vi "PianoTest 8 channel.vi"() -> ()   [LabVIEW 2013]
uses:
  <vilib>/rvi/Emulation/niFpgaSctlEmulationGetInTimedLoop.vi
  <vilib>/rvi/Emulation/niFpgaEmulationReportErrorSimple.vi
  <vilib>/rvi/Emulation/niFpgaGetClockAttributes.vi
  <vilib>/rvi/eio/common/nirviEmuTemplateMethod_errors.vi
  <vilib>/rvi/Emulation/niFpgaCriticalErrorInLSC.vi
  <vilib>/eio/EIONode/EIONode.xnode
panel:
  in  "PWM1 Period (us)":fxp<+/-,20,16>=130.0
  in  "PWM1 Duty Cycle %":fxp<+/-,20,16>=100.0
  in  "Play":bool
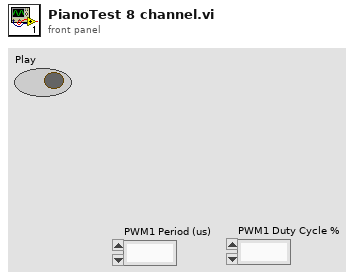
[diagram p1: front panel]
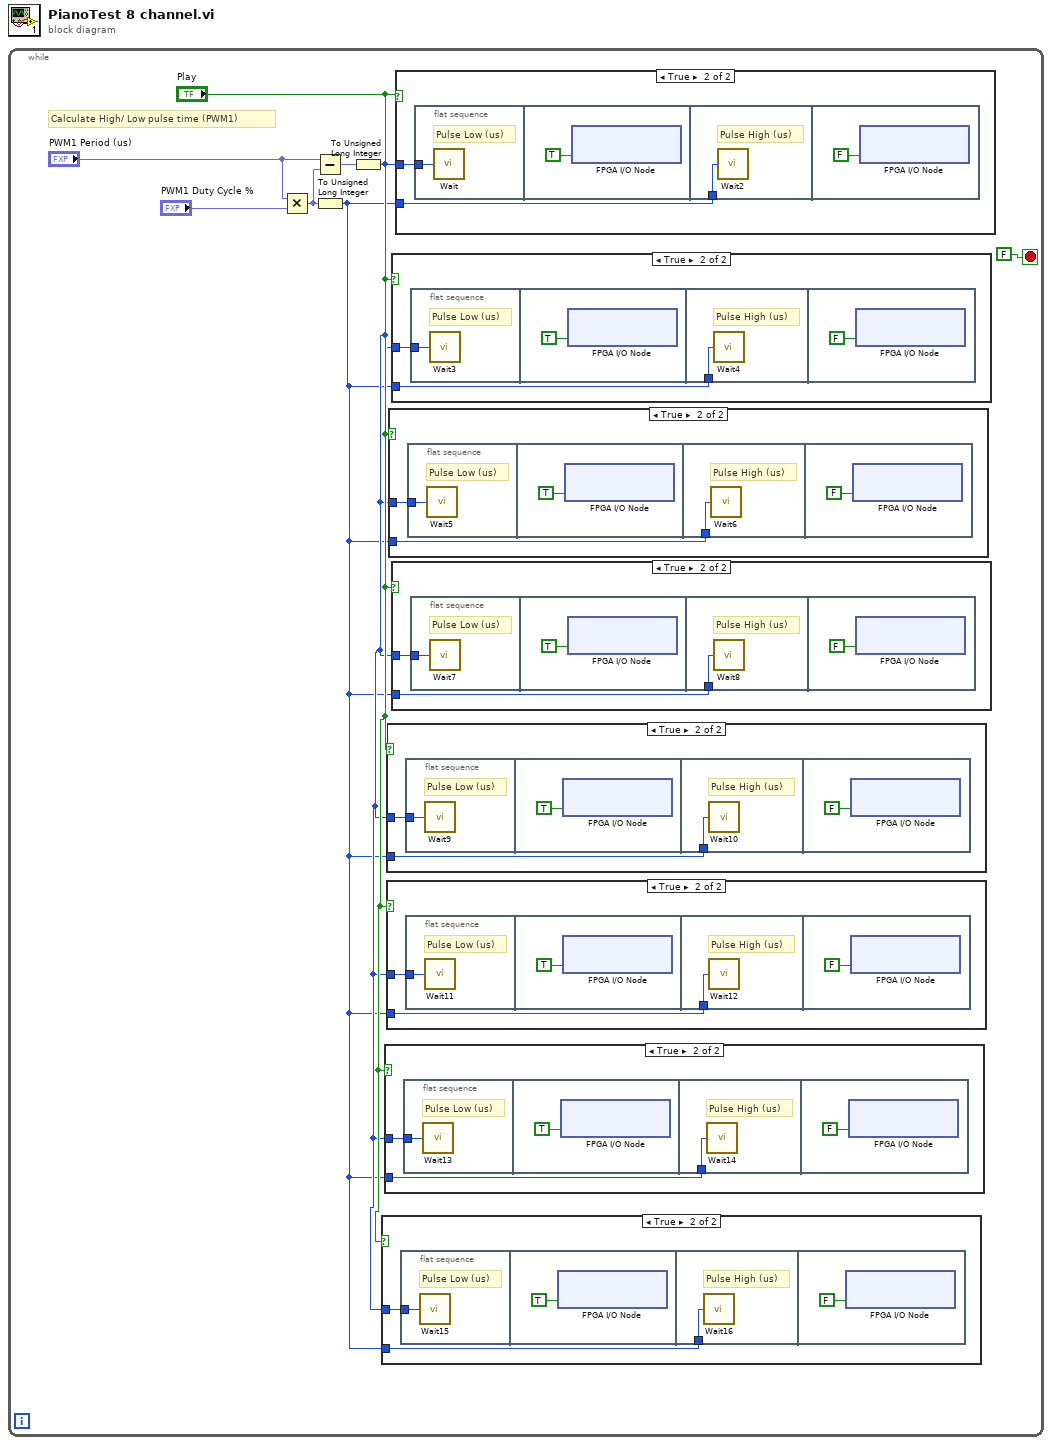
[diagram p0: block diagram]
diagram:
  n1 = while {
    stop <- FALSE stop-if-true
    # "Calculate High/ Low pulse time (PWM1)"
    n2 = Multiply(x="PWM1 Period (us)", y="PWM1 Duty Cycle %") -> (x*y=w7:fxp<+/-,40,32>)
    n3 = Subtract(x="PWM1 Period (us)", y=w7) -> (x-y=w4:fxp<+/-,40,32>)
    n4 = To Unsigned Long Integer(number=w7) -> (unsigned 32bit integer=w1:u32)
    n5 = To Unsigned Long Integer(number=w4) -> (unsigned 32bit integer=w2:u32)
    n6 = case shown="True" "Play" {
      tunnel: w1 -> [_ w10]
      tunnel: w2 -> [_ w9]
      frame False {
      }
      frame True {
        n7 = flat-sequence {
          tunnel: w9 -> [w11]
          tunnel: w10 -> [w13]
          frame #0 {
            # "Pulse Low (us)"
            n8 = call "Wait15"("Count(uSec)"=w11) -> ()  [unwired: 1 out]
          }
          frame #1 {
            n9 = xnode "FPGA I/O Node"("Mod1/DO7"=TRUE ("PWM 1T")) -> ()  [unwired: 1 in, 1 out]
          }
          frame #2 {
            # "Pulse High (us)"
            n10 = call "Wait16"("Count(uSec)"=w13) -> ()  [unwired: 1 out]
          }
          frame #3 {
            n11 = xnode "FPGA I/O Node"("Mod1/DO7"=FALSE ("PWM 1T")) -> ()  [unwired: 1 in, 1 out]
          }
        }
      }
    }
    n12 = case shown="True" "Play" {
      tunnel: w1 -> [_ w16]
      tunnel: w2 -> [_ w15]
      frame False {
      }
      frame True {
        n13 = flat-sequence {
          tunnel: w15 -> [w17]
          tunnel: w16 -> [w19]
          frame #0 {
            # "Pulse Low (us)"
            n14 = call "Wait13"("Count(uSec)"=w17) -> ()  [unwired: 1 out]
          }
          frame #1 {
            n15 = xnode "FPGA I/O Node"("Mod1/DO6"=TRUE ("PWM 1T")) -> ()  [unwired: 1 in, 1 out]
          }
          frame #2 {
            # "Pulse High (us)"
            n16 = call "Wait14"("Count(uSec)"=w19) -> ()  [unwired: 1 out]
          }
          frame #3 {
            n17 = xnode "FPGA I/O Node"("Mod1/DO6"=FALSE ("PWM 1T")) -> ()  [unwired: 1 in, 1 out]
          }
        }
      }
    }
    n18 = case shown="True" "Play" {
      tunnel: w1 -> [_ w28]
      tunnel: w2 -> [_ w27]
      frame False {
      }
      frame True {
        n19 = flat-sequence {
          tunnel: w27 -> [w29]
          tunnel: w28 -> [w31]
          frame #0 {
            # "Pulse Low (us)"
            n20 = call "Wait9"("Count(uSec)"=w29) -> ()  [unwired: 1 out]
          }
          frame #1 {
            n21 = xnode "FPGA I/O Node"("Mod1/DO4"=TRUE ("PWM 1T")) -> ()  [unwired: 1 in, 1 out]
          }
          frame #2 {
            # "Pulse High (us)"
            n22 = call "Wait10"("Count(uSec)"=w31) -> ()  [unwired: 1 out]
          }
          frame #3 {
            n23 = xnode "FPGA I/O Node"("Mod1/DO4"=FALSE ("PWM 1T")) -> ()  [unwired: 1 in, 1 out]
          }
        }
      }
    }
    n24 = case shown="True" "Play" {
      tunnel: w1 -> [_ w22]
      tunnel: w2 -> [_ w21]
      frame False {
      }
      frame True {
        n25 = flat-sequence {
          tunnel: w21 -> [w23]
          tunnel: w22 -> [w25]
          frame #0 {
            # "Pulse Low (us)"
            n26 = call "Wait11"("Count(uSec)"=w23) -> ()  [unwired: 1 out]
          }
          frame #1 {
            n27 = xnode "FPGA I/O Node"("Mod1/DO5"=TRUE ("PWM 1T")) -> ()  [unwired: 1 in, 1 out]
          }
          frame #2 {
            # "Pulse High (us)"
            n28 = call "Wait12"("Count(uSec)"=w25) -> ()  [unwired: 1 out]
          }
          frame #3 {
            n29 = xnode "FPGA I/O Node"("Mod1/DO5"=FALSE ("PWM 1T")) -> ()  [unwired: 1 in, 1 out]
          }
        }
      }
    }
    n30 = case shown="True" "Play" {
      tunnel: w1 -> [_ w40]
      tunnel: w2 -> [_ w39]
      frame False {
      }
      frame True {
        n31 = flat-sequence {
          tunnel: w39 -> [w41]
          tunnel: w40 -> [w43]
          frame #0 {
            # "Pulse Low (us)"
            n32 = call "Wait5"("Count(uSec)"=w41) -> ()  [unwired: 1 out]
          }
          frame #1 {
            n33 = xnode "FPGA I/O Node"("Mod1/DO2"=TRUE ("PWM 1T")) -> ()  [unwired: 1 in, 1 out]
          }
          frame #2 {
            # "Pulse High (us)"
            n34 = call "Wait6"("Count(uSec)"=w43) -> ()  [unwired: 1 out]
          }
          frame #3 {
            n35 = xnode "FPGA I/O Node"("Mod1/DO2"=FALSE ("PWM 1T")) -> ()  [unwired: 1 in, 1 out]
          }
        }
      }
    }
    n36 = case shown="True" "Play" {
      tunnel: w1 -> [_ w46]
      tunnel: w2 -> [_ w45]
      frame False {
      }
      frame True {
        n37 = flat-sequence {
          tunnel: w45 -> [w47]
          tunnel: w46 -> [w49]
          frame #0 {
            # "Pulse Low (us)"
            n38 = call "Wait3"("Count(uSec)"=w47) -> ()  [unwired: 1 out]
          }
          frame #1 {
            n39 = xnode "FPGA I/O Node"("Mod1/DO1"=TRUE ("PWM 1T")) -> ()  [unwired: 1 in, 1 out]
          }
          frame #2 {
            # "Pulse High (us)"
            n40 = call "Wait4"("Count(uSec)"=w49) -> ()  [unwired: 1 out]
          }
          frame #3 {
            n41 = xnode "FPGA I/O Node"("Mod1/DO1"=FALSE ("PWM 1T")) -> ()  [unwired: 1 in, 1 out]
          }
        }
      }
    }
    n42 = case shown="True" "Play" {
      tunnel: w1 -> [_ w34]
      tunnel: w2 -> [_ w33]
      frame False {
      }
      frame True {
        n43 = flat-sequence {
          tunnel: w33 -> [w35]
          tunnel: w34 -> [w37]
          frame #0 {
            # "Pulse Low (us)"
            n44 = call "Wait7"("Count(uSec)"=w35) -> ()  [unwired: 1 out]
          }
          frame #1 {
            n45 = xnode "FPGA I/O Node"("Mod1/DO3"=TRUE ("PWM 1T")) -> ()  [unwired: 1 in, 1 out]
          }
          frame #2 {
            # "Pulse High (us)"
            n46 = call "Wait8"("Count(uSec)"=w37) -> ()  [unwired: 1 out]
          }
          frame #3 {
            n47 = xnode "FPGA I/O Node"("Mod1/DO3"=FALSE ("PWM 1T")) -> ()  [unwired: 1 in, 1 out]
          }
        }
      }
    }
    n48 = case shown="True" "Play" {
      tunnel: w1 -> [_ w52]
      tunnel: w2 -> [_ w51]
      frame False {
      }
      frame True {
        n49 = flat-sequence {
          tunnel: w51 -> [w53]
          tunnel: w52 -> [w55]
          frame #0 {
            # "Pulse Low (us)"
            n50 = call "Wait"("Count(uSec)"=w53) -> ()  [unwired: 1 out]
          }
          frame #1 {
            n51 = xnode "FPGA I/O Node"("Mod1/DO0"=TRUE ("PWM 1T")) -> ()  [unwired: 1 in, 1 out]
          }
          frame #2 {
            # "Pulse High (us)"
            n52 = call "Wait2"("Count(uSec)"=w55) -> ()  [unwired: 1 out]
          }
          frame #3 {
            n53 = xnode "FPGA I/O Node"("Mod1/DO0"=FALSE ("PWM 1T")) -> ()  [unwired: 1 in, 1 out]
          }
        }
      }
    }
  }
